vi "Create Datafile Path.vi"(1 "Position":u8=1 min=1, 2 "Rack":u8=1 min=1, 3 "System":u8=1 min=1, 4 "Data Directory":path=path "c:/cmf/data") -> (0 "Data Path":path)   [LabVIEW 2021]
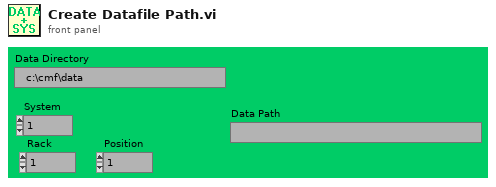
[diagram p1: front panel]
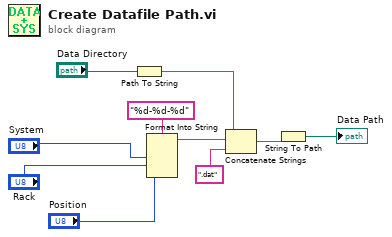
[diagram p0: block diagram]
diagram:
  n1 = Path To String(path="Data Directory") -> (string=w1:string)
  n2 = Format Into String(format string="%d-%d-%d" ("Format String"), "System", "Rack", "Position") -> (resulting string=w9:string)  [unwired: 2 in, 1 out]
  n3 = Concatenate Strings(w1, w9, ".dat" ("Substring")) -> (w7:string)
  n4 = String To Path(string=w7) -> (path=→"Data Path":path)
